vi "Coral Teleop Handler.vi"() -> ()   [LabVIEW 2023]
uses:
  Teleop Util/Coral States.ctl
  Teleop Util/Scoring Setpoint.ctl
  Teleop Util/Scoring Levels.ctl
  <vilib>/Rock Robotics/WPI/Joystick/XBox Axes Indexer.ctl
  <vilib>/Rock Robotics/WPI/Joystick/XBox Buttons Indexer.ctl
  Coral/Implementation/Coral Operations.ctl
  02b96f5f-4aa0-4050-af39-5bf6ce57af74.vi
  ac154037-dd92-4d3b-9487-38ca34f15abd.vi
  41f243a3-b476-470d-886f-9ab9dadf628b.vi
  d73daf83-586d-4580-b12c-c6ead0d00ab0.vi
  <vilib>/Rock Robotics/WPI/Utilities/WPI_GetSetVariantRefNum.vi
  Framework/Robot Global Data.vi
panel:
  in  "Left Rumble":sgl
  out "Final Setpoint":T1=enum."L2"
  in  "Scoring Setpoint":T2=[enum."Trough", enum."L2", enum."L3", enum."L4"]
  out "testing states bz":T3
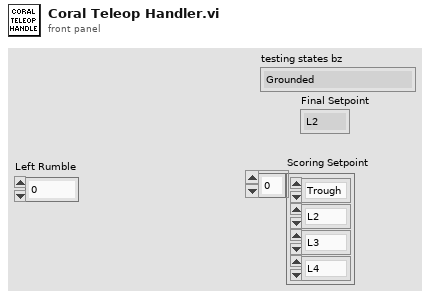
[diagram p1: front panel]
types:
  T1 = typedef "Scoring Levels.ctl" = enum16{"Trough", "L2", "L3", "L4", "Default"}
  T2 = typedef "Scoring Setpoint.ctl" = enum16{"Trough", "L2", "L3", "L4"}[]
  T3 = typedef "Coral States.ctl" = enum16{"Grounded", "Coral Intake", "Scoring Sequence", "Hold Position", "Score", "Manual Override", "Climb Safety Mode"}
  T4 = typedef "XBox Buttons Indexer.ctl" = enum16{"A", "B", "X", "Y", "Left Bumper", "Right Bumper", "Back", "Start", "Left Joystick", "Right Joystick"}
  T5 = typedef "XBox Axes Indexer.ctl" = enum16{"Left X", "Left Y", "Left Trigger", "Right Trigger", "Right X", "Right Y"}
  T6 = typedef "WPI_JoystickDevRef.ctl" = cluster{"Device":T7}
  T7 = typedef "WPI_JoystickDeviceEnum.ctl" = enum16{"USB 0", "USB 1", "USB 2", "USB 3", "USB 4", "USB 5"}
  T8 = typedef "Coral Operations.ctl" = enum16{"Reserve", "Read Current", "Immediate", "Calibrate"}
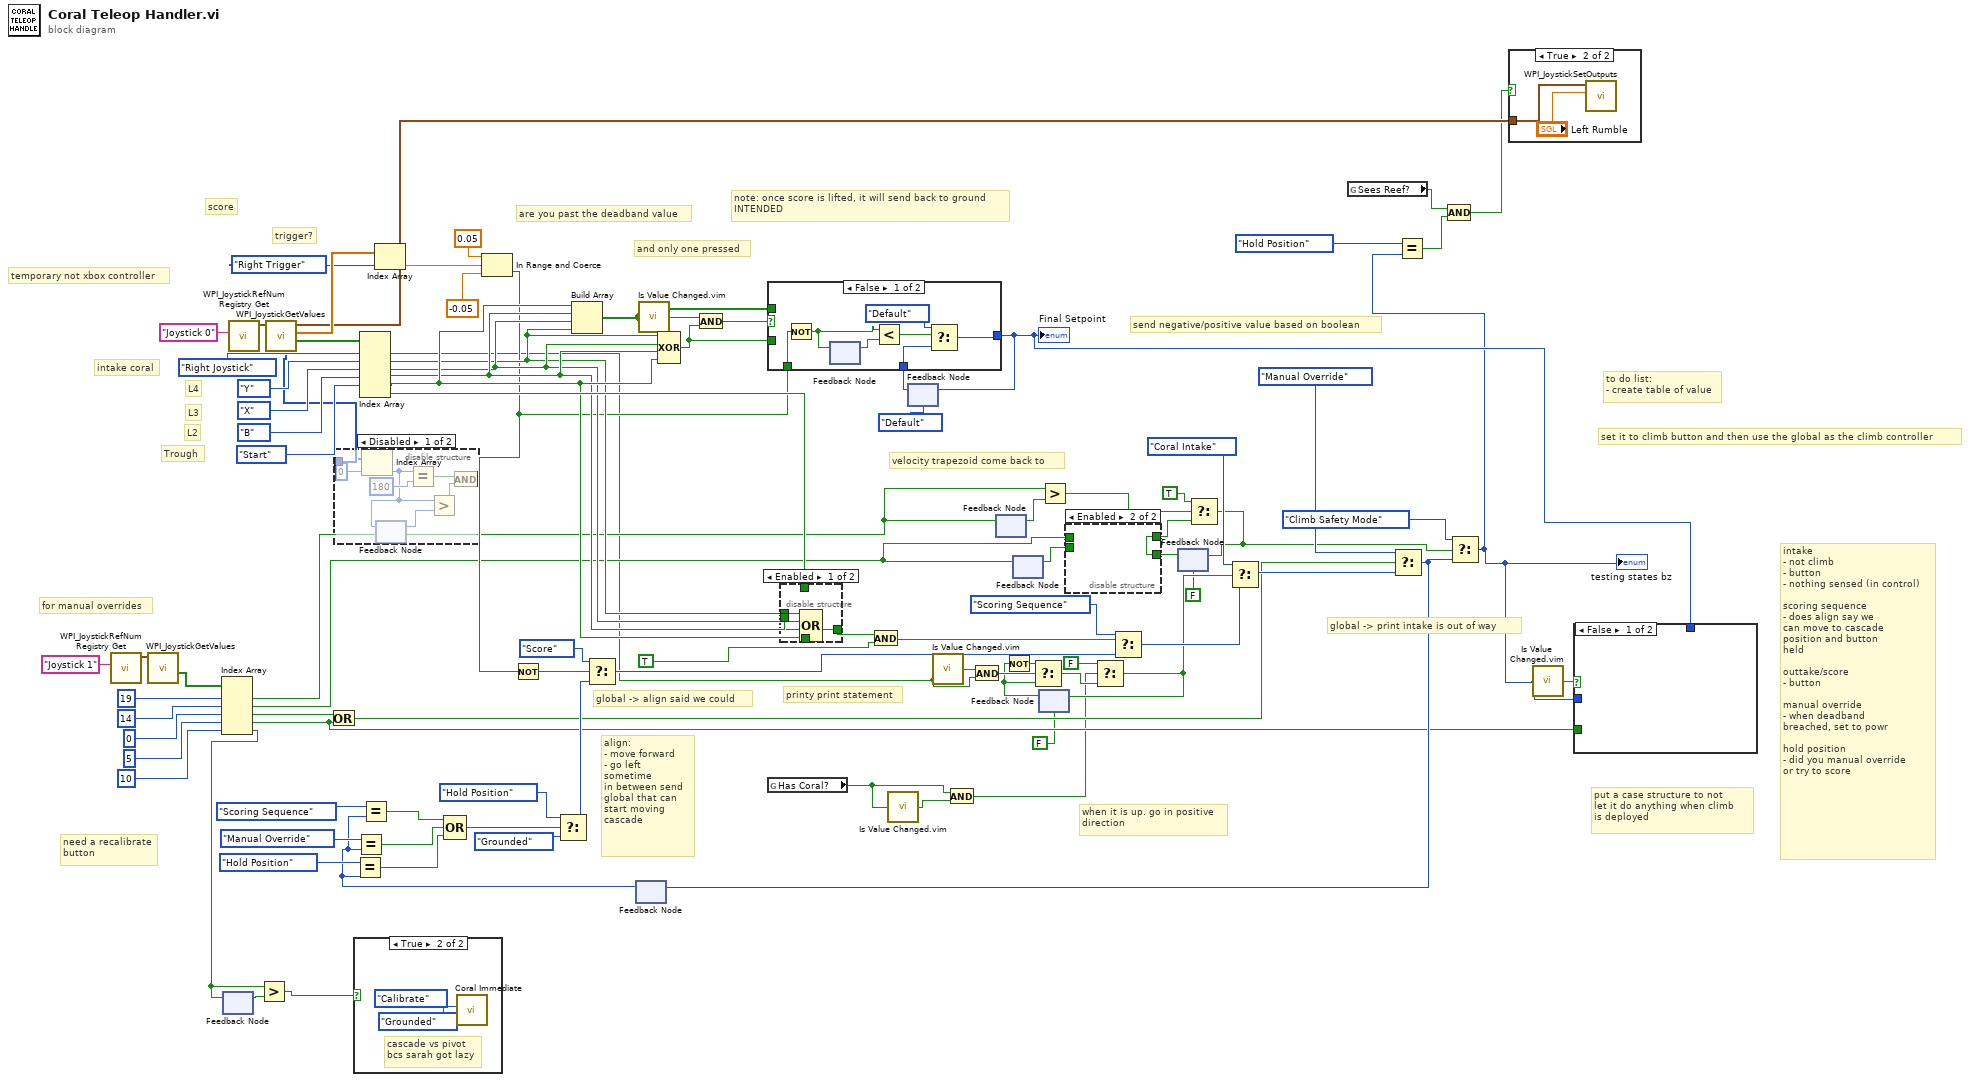
[diagram p0: block diagram]
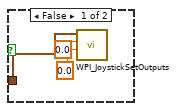
[diagram p2: hidden frame]
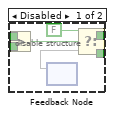
[diagram p4: hidden frame]
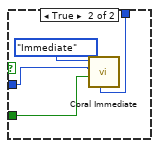
[diagram p6: hidden frame]
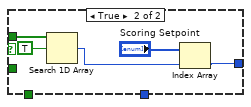
[diagram p8: hidden frame]
diagram:
  # "score"
  # "when it is up. go in positive\ndirection"
  # "send negative/positive value based on boolean"
  # "global -> print intake is out of way"
  # "printy print statement"
  # "set it to climb button and then use the global as the climb controller"
  # "put a case structure to not\nlet it do anything when climb \nis deployed"
  # "note: once score is lifted, it will send back to ground\nINTENDED"
  # "velocity trapezoid come back to"
  # "intake coral"
  # "and only one pressed"
  # "to do list:\n- create table of value"
  # "Trough"
  # "L2"
  # "L3"
  # "L4"
  # "need a recalibrate\nbutton"
  # "align:\n- move forward\n- go left \nsometime \nin between send \nglobal that can \nstart moving \ncascade"
  # "global -> align said we could"
  # "are you past the deadband value"
  # "trigger?"
  # "temporary not xbox controller"
  # "intake\n- not climb\n- button\n- nothing sensed (in control)\n\nscoring sequence\n- does align say we\ncan move to cascade\nposition and button\nheld\n\nouttake/score\n- button\n\nmanual override\n- when deadband\nbreached, set to powr\n\nhold position\n- did you manual override\nor try to score"
  # "for manual overrides"
  n1 = call <vilib>:"WPI_JoystickRefNum Registry Get.vi"("refnum name"="Joystick 1") -> ("JoystickDevRef"=w91:T6)  [unwired: 1 in, 9 out]
  n2 = call <vilib>:"WPI_JoystickGetValues.vi"("JoystickDevRef"=w91) -> ("Buttons"=w89:bool[])  [unwired: 6 in, 4 out]
  n3 = Index Array(array=w89, index #1=19 ("index"), index #2=14 ("index"), index #3=0 ("index"), index #4=5 ("index"), index #5=10 ("index")) -> (element #1=w27:bool, element #2=w28:bool, element #3=w37:bool, element #4=w36:bool, element #5=w31:bool)
  n4 = feedback-in #1(w31) -> ()
  n5 = feedback #1() -> (w44:bool)  [unwired: 1 in]
  n6 = call <vilib>:"WPI_JoystickRefNum Registry Get.vi"("refnum name"="Joystick 0") -> ("JoystickDevRef"=w94:T6)  [unwired: 1 in, 9 out]
  n7 = Greater?(x=w31, y=w44) -> (0:w9:bool)
  n8 = call <vilib>:"WPI_JoystickGetValues.vi"("JoystickDevRef"=w94) -> ("Buttons"=w92:bool[], "Axes"=w76:dbl[], "JoystickDevRef"=w8:T6, "POVs"=w10:i16[])  [unwired: 6 in, 1 out]
  n9 = Or(x=w37, y=w36) -> (x .or. y?=w35:bool)
  n10 = disable-structure shown="Disabled" {
    disable-tunnel: w10 -> [w101 _]
    frame Disabled {
      n11 = Index Array(array=w101, index=0) -> (element=w98:i16)
      n12 = feedback #2() -> (w97:i16)  [unwired: 1 in]
      n13 = feedback-in #2(w98) -> ()
      n14 = Equal?(x=w98, y=i16 180) -> (x = y?=w95:bool)
      n15 = Greater?(x=w98, y=w97) -> (0:w96:bool)
      n16 = And(x=w95, y=w96) -> ()  [unwired: 1 out]
    }
    frame Enabled {
    }
  }
  n17 = case shown="True" w9 {
    frame False {
    }
    frame True {
      # "cascade vs pivot\nbcs sarah got lazy"
      n18 = call "Coral Immediate.vi"("Coral States"=Coral_States."Grounded", "Operation"=Coral_Operations."Calibrate") -> ()  [unwired: 9 in, 1 out]
    }
  }
  n19 = Index Array(array=w92, index #1=XBox_Buttons_Indexer."Right Joystick" ("XBox Buttons"), index #2=XBox_Buttons_Indexer."Y" ("XBox Buttons"), index #3=XBox_Buttons_Indexer."X" ("XBox Buttons"), index #4=XBox_Buttons_Indexer."B" ("XBox Buttons"), index #5=XBox_Buttons_Indexer."Start" ("XBox Buttons")) -> (element #1=w22:bool, element #2=w49:bool, element #3=w50:bool, element #4=w51:bool, element #5=w52:bool, element #6=w53:bool)  [unwired: 1 in]
  n20 = Index Array(array=w76, index=XBox_Axes_Indexer."Right Trigger" ("XBox Axes")) -> (element=w73:dbl)
  n21 = In Range and Coerce(upper limit=0.05 ("lower limit"), x=w73, lower limit=-0.05) -> (In Range?=w38:bool)  [unwired: 1 out]
  n22 = Not(x=w38) -> (.not. x?=w17:bool)
  n23 = Build Array(w52, w51, w50, w49) -> (w65:bool[])
  n24 = feedback #3() -> (w54:T3)  [unwired: 1 in]
  n25 = Equal?(x=Coral_States."Hold Position", y=w54) -> (x = y?=w57:bool)
  n26 = Equal?(x=Coral_States."Manual Override", y=w54) -> (x = y?=w58:bool)
  n27 = Equal?(x=Coral_States."Scoring Sequence", y=w54) -> (x = y?=w59:bool)
  n28 = Compound Arithmetic op=OR(w59, w58, w57) -> (w56:bool)
  n29 = Select(t=Coral_States."Hold Position", s=w56, f=Coral_States."Grounded") -> (s? t:f=w87:T3)
  n30 = Select(t=Coral_States."Score", s=w17, f=w87) -> (s? t:f=w85:T3)
  n31 = call "Is Value Changed.vim"("value"=w65) -> ("changed or first call?"=w66:bool)
  n32 = Compound Arithmetic op=XOR(w49, w50, w51, w52) -> (w63:bool)
  n33 = And(x=w66, y=w63) -> (x .and. y?=w64:bool)
  n34 = global read "Robot Global Data.vi" "Has Coral?"() -> (w1:bool)
  n35 = disable-structure shown="Enabled" {
    disable-tunnel: w49 -> [w108 _]
    disable-tunnel: w50 -> [w107 _]
    disable-tunnel: w51 -> [w106 _]
    disable-tunnel: w52 -> [w105 _]
    disable-tunnel: [w104 w109] -> w61
    disable-tunnel: w53 -> [_ w109]
    frame Enabled {
      n36 = Compound Arithmetic op=OR(w108, w107, w106, w105) -> (w104:bool)
    }
    frame Disabled {
    }
  }
  n37 = And(x=w61, y=TRUE) -> (x .and. y?=w62:bool)
  n38 = call "Is Value Changed.vim"("value"=w1) -> ("changed or first call?"=w16:bool)
  n39 = feedback #4(Scoring_Levels."Default" ("t")) -> (w48:T1)
  n40 = case shown="False" w64 {
    tunnel: w65 -> [_ w121]
    tunnel: w63 -> [_ _]
    tunnel: w48 -> [w113 _]
    tunnel: w38 -> [w115 _]
    tunnel: [w111 w117] -> w7
    frame False {
      n41 = Not(x=w115) -> (.not. x?=w110:bool)
      n42 = feedback-in #5(w110) -> ()
      n43 = feedback #5() -> (w114:bool)  [unwired: 1 in]
      n44 = Less?(x=w110, y=w114) -> (x < y?=w116:bool)
      n45 = Select(t=Scoring_Levels."Default", s=w116, f=w113) -> (s? t:f=w111:T1)
    }
    frame True {
      n46 = Search 1D Array(1D array=w121, element=TRUE) -> (index of element=w120:i32)  [unwired: 1 in]
      n47 = Index Array(array="Scoring Setpoint", index=w120) -> (element=w117:enum16{"Trough", "L2", "L3", "L4"})
    }
  }
  "Final Setpoint" <- w7
  n48 = feedback-in #4(w7) -> ()
  n49 = call "Is Value Changed.vim"("value"=w22) -> ("changed or first call?"=w25:bool)
  n50 = And(x=w1, y=w16) -> (x .and. y?=w15:bool)
  n51 = And(x=w25, y=w22) -> (x .and. y?=w26:bool)
  n52 = feedback-in #6(w27) -> ()
  n53 = feedback #6() -> (w43:bool)  [unwired: 1 in]
  n54 = feedback #7() -> (w40:bool)  [unwired: 1 in]
  n55 = feedback-in #7(w28) -> ()
  n56 = feedback #8(FALSE) -> (w24:bool)
  n57 = Not(x=w24) -> (.not. x?=w21:bool)
  n58 = Select(t=w21, s=w26, f=w24) -> (s? t:f=w19:bool)
  n59 = Greater?(x=w27, y=w43) -> (0:w42:bool)
  n60 = Select(t=FALSE, s=w15, f=w19) -> (s? t:f=w20:bool)
  n61 = feedback-in #8(w20) -> ()
  n62 = Select(t=Coral_States."Scoring Sequence", s=w62, f=w85) -> (s? t:f=w84:T3)
  n63 = feedback #9(FALSE) -> (w11:bool)
  n64 = disable-structure shown="Enabled" {
    disable-tunnel: [w127 w128] -> w14
    disable-tunnel: w40 -> [w125 _]
    disable-tunnel: w28 -> [w122 _]
    disable-tunnel: w11 -> [_ w128]
    frame Disabled {
      n65 = Greater?(x=w122, y=w125) -> (0:w124:bool)
      n66 = feedback #10() -> (w126)  [unwired: 1 in]
      n67 = feedback-in #10() -> ()  [unwired: 1 out]
      n68 = Select(t=FALSE, s=w124, f=w126) -> (s? t:f=w127:bool)
    }
    frame Enabled {
    }
  }
  n69 = Select(t=TRUE, s=w42, f=w14) -> (s? t:f=w13:bool)
  n70 = feedback-in #9(w13) -> ()
  n71 = Select(t=Coral_States."Coral Intake", s=w20, f=w84) -> (s? t:f=w83:T3)
  n72 = global read "Robot Global Data.vi" "Sees Reef?"() -> (w4:bool)
  n73 = Select(t=Coral_States."Manual Override", s=w35, f=w83) -> (s? t:f=w46:T3)
  n74 = feedback-in #3(w46) -> ()
  n75 = Select(t=Coral_States."Climb Safety Mode", s=w13, f=w46) -> (s? t:f=w6:T3)
  "testing states bz" <- w6
  n76 = Equal?(x=Coral_States."Hold Position", y=w6) -> (x = y?=w2:bool)
  n77 = Compound Arithmetic op=AND(w4, w2) -> (w3:bool)
  n78 = case shown="True" w3 {
    tunnel: w8 -> [w131 w133]
    frame False {
      n79 = call <vilib>:"WPI_JoystickSetOutputs.vi"("Right Rumble"=sgl 0.0, "Left Rumble"=sgl 0.0, "JoystickDevRef"=w131) -> ()  [unwired: 7 in, 2 out]
    }
    frame True {
      n80 = call <vilib>:"WPI_JoystickSetOutputs.vi"("Left Rumble"="Left Rumble", "JoystickDevRef"=w133) -> ()  [unwired: 8 in, 2 out]
    }
  }
  n81 = call "Is Value Changed.vim"("value"=w6) -> ("changed or first call?"=w47:bool)
  n82 = case shown="False" w47 {
    tunnel: w7 -> [_ w136]
    tunnel: w6 -> [_ w135]
    tunnel: w36 -> [_ w134]
    frame False {
    }
    frame True {
      n83 = call "Coral Immediate.vi"("Setpoint State"=w136, "Confirm or Negate"=w134, "Coral States"=w135, "Operation"=Coral_Operations."Immediate") -> ()  [unwired: 7 in, 1 out]
    }
  }
